vi "DAQmx Read (Digital 1D U8 1Chan NSamp).vi"(0 "task/channels in":refnum<k21>, 7 "number of samples per channel":i32=-1, 9 "timeout":dbl=10.0 format="%0.2f", 11 "error in":errorcluster) -> (4 "task out":refnum<k21>, 6 "data":u8[](array[numeric]), 15 "error out":errorcluster)   [LabVIEW 2022 SP3]
doc: "Reads one or more 8-bit unsigned integer samples from a task that contains a single digital input channel. Use an instance that reads 8-bit unsigned integers for devices with up to eight lines per port."
uses:
  nilvaiu.dll
panel:
  # "sample #"
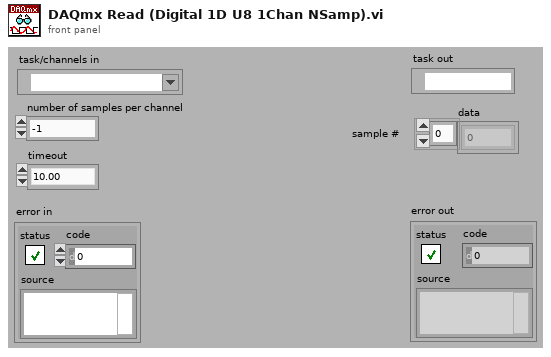
[diagram p1: front panel]
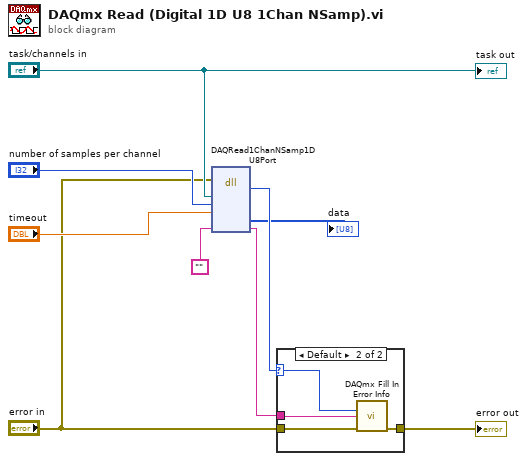
[diagram p0: block diagram]
diagram:
  n1 = dll-call lib="nilvaiu.*" fn="DAQRead1ChanNSamp1DU8Port"(error in="error in", "taskID"="task/channels in", "samplesPerChannel"="number of samples per channel", "timeout"="timeout", "extendedErrorInfo"="") -> ("return type"=w7:i32, "data"=→"data":u8[], "extendedErrorInfo"=w3:string)  [unwired: 5 in, 3 out]
  n2 = case shown="Default" w7 {
    selector: w7 -> [_ w12]
    tunnel: "error in" -> [w10 w14]
    tunnel: [w10 w13] -> w9
    tunnel: w3 -> [_ w11]
    frame 0 {
    }
    frame Default {
      n3 = call "DAQmx Fill In Error Info.vi"("status code"=w12, "extended error info"=w11, "error in"=w14) -> ("error out"=w13:errorcluster)  [unwired: 1 in, 11 out]
    }
  }
  "error out" <- w9
  "task out" <- "task/channels in"
